vi "Girouette.vi"(8 "girouette":dbl) -> (0 "Direction de la Girouette":string, 1 "Boussole":i32(knob) scale=0.0..8.0)   [LabVIEW 2017]
panel:
  out "Sortie du Capteur":dbl
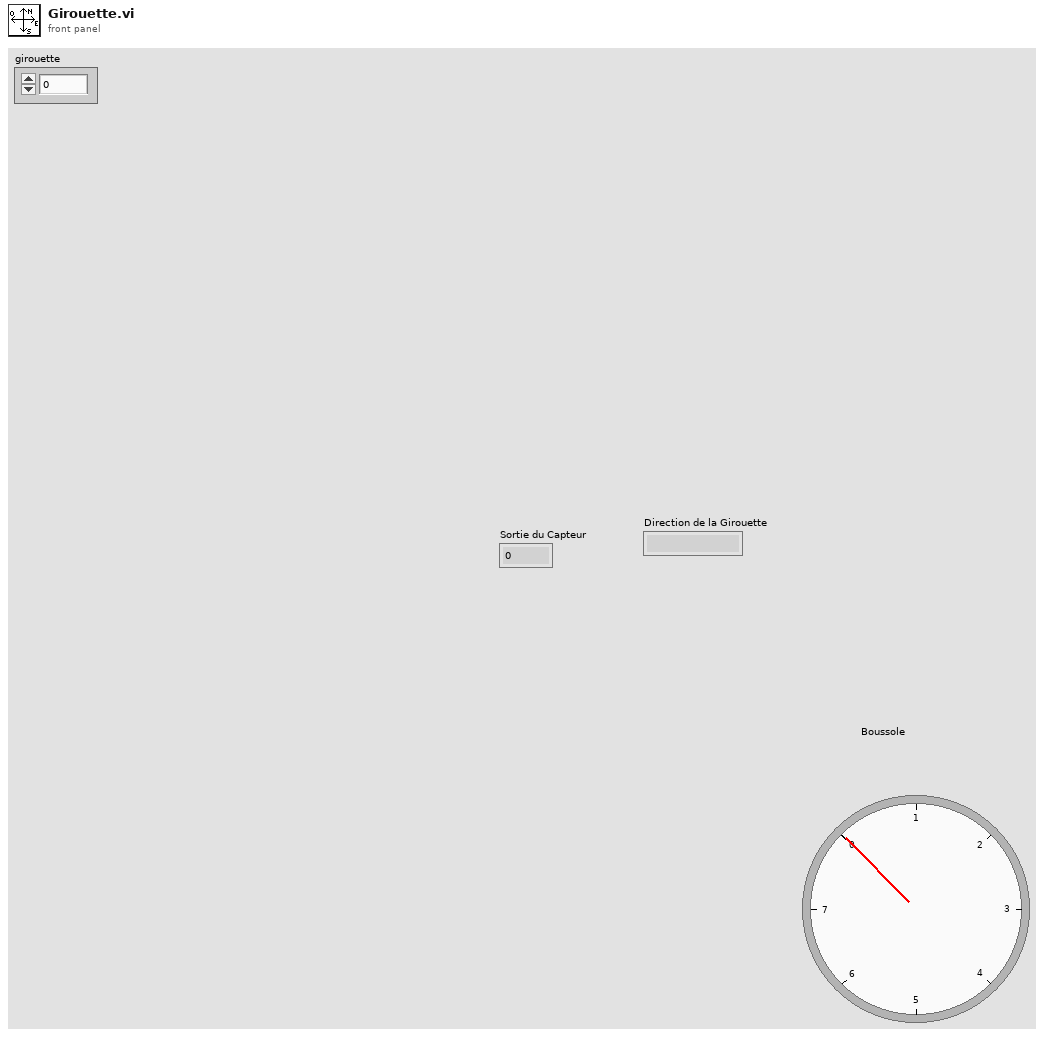
[diagram p1: front panel]
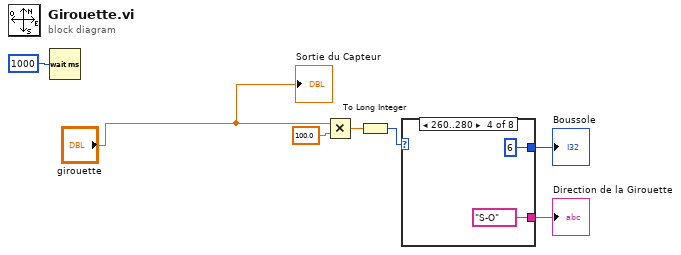
[diagram p0: block diagram]
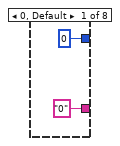
[diagram p2: hidden frame]
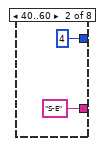
[diagram p3: hidden frame]
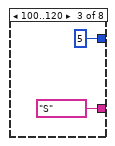
[diagram p4: hidden frame]
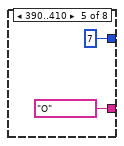
[diagram p5: hidden frame]
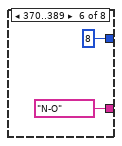
[diagram p6: hidden frame]
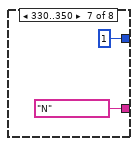
[diagram p7: hidden frame]
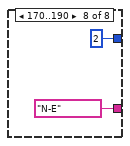
[diagram p8: hidden frame]
diagram:
  n1 = Wait (ms)(milliseconds to wait=u32 1000 ("attente (ms)")) -> ()  [unwired: 1 out]
  n2 = Multiply(x="girouette", y=100.0) -> (x*y=w5:dbl)
  n3 = To Long Integer(number=w5) -> (32bit integer=w4:i32)
  n4 = case shown="260..280" w4 {
    tunnel: [0 4 5 6 7 8 1 2] -> w2
    tunnel: ["0" "S-E" "S" "S-O" "O" "N-O" "N" "N-E"] -> w3
    frame 0, Default {
    }
    frame 40..60 {
    }
    frame 100..120 {
    }
    frame 260..280 {
    }
    frame 390..410 {
    }
    frame 370..389 {
    }
    frame 330..350 {
    }
    frame 170..190 {
    }
  }
  "Direction de la Girouette" <- w3
  "Boussole" <- w2
  "Sortie du Capteur" <- "girouette"
